vi "getDeconMatrixSize.vi"(8 "error in (no error)":errorcluster, 11 "LaguerreDeconClass in":refnum<class "LaguerreDeconEngineClass.lvclass">) -> (0 "error out":errorcluster, 2 "data Matrix Szie":T1, 3 "LaguerreDeconClass out":refnum<class "LaguerreDeconEngineClass.lvclass">)   [LabVIEW 2024, in "LaguerreDeconEngineClass.lvclass"]
uses:
  LaguerreDeconEngineClass.lvclass
  LaguerreDeconEngineClass.lvclass/LaguerreDeconEngineClass.ctl
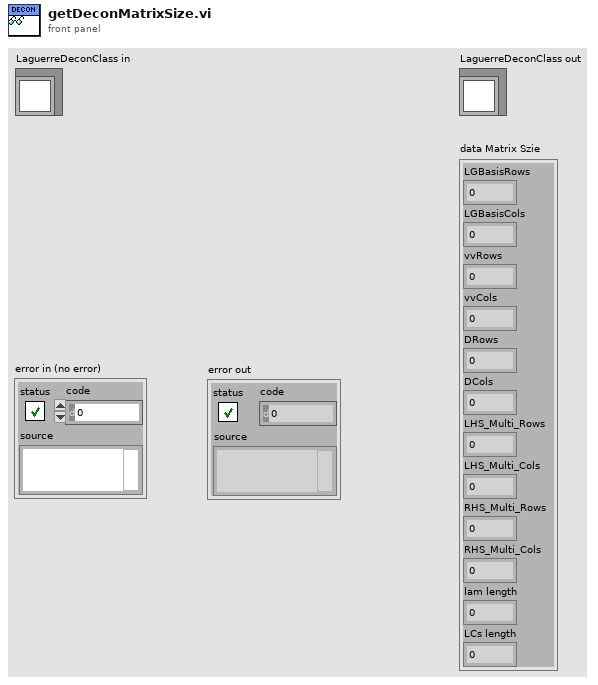
[diagram p1: front panel]
types:
  T1 = cluster{"LGBasisRows":u32, "LGBasisCols":u32, "vvRows":u32, "vvCols":u32, "DRows":u32, "DCols":u32, "LHS_Multi_Rows":u32, "LHS_Multi_Cols":u32, "RHS_Multi_Rows":u32, "RHS_Multi_Cols":u32, "lam length":u32, "LCs length":u32}
  T2 = cluster{"LGBasisRows":u64, "LGBasisCols":u64, "vvRows":u64, "vvCols":u64, "DRows":u64, "DCols":u64, "LHS_Multi_Rows":u64, "LHS_Multi_Cols":u64, "RHS_Multi_Rows":u64, "RHS_Multi_Cols":u64, "lam length":u64, "LCs length":u64}
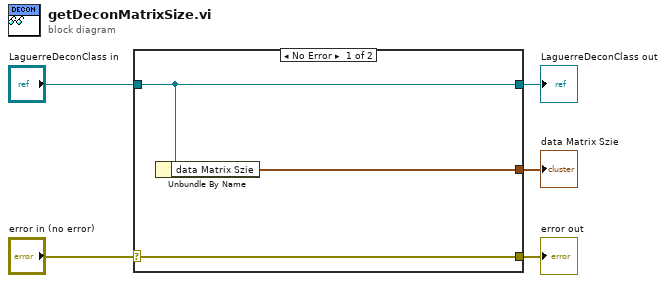
[diagram p0: block diagram]
diagram:
  n1 = case shown="No Error" "error in (no error)" {
    selector: "error in (no error)" -> [w8 w9]
    tunnel: [w8 w9] -> w4
    tunnel: [w7 w10] -> w2
    tunnel: "LaguerreDeconClass in" -> [w7 w10]
    tunnel: [w6 _] -> w1
    frame No Error {
      n2 = Unbundle By Name(w7) -> ("data Matrix Szie"=w6:T2)
    }
    frame Error {
    }
  }
  "error out" <- w4
  "LaguerreDeconClass out" <- w2
  "data Matrix Szie" <- w1
